vi "dfd_Cosine Modulation.vi"(6 "fs in [Hz]":dbl=1.0, 7 "number of bands":i32=4, 8 "error in (no error)":errorcluster, 11 "h":dbl[](array[numeric])) -> (0 "error out":errorcluster, 2 "synthesis bank":T1[](array[typedef]) {"mMRate_SumWl" min=1 max=32 step=1; "mMRate_InputIwl" min=1 max=32 step=1; "mMRate_GainWl" min=1 max=32 step=1; "mMRate_OutputWl" min=1 max=32 step=1; "mMRate_InputWl" min=1 max=32 step=1; "mMRate_CoefWl" min=1 max=32 step=1; "mMRate_Mode" items=["Default"=-1, "No Rate Change"=0, "Interpolation"=1, "Decimation"=2, "Interpolated"=3, "Rational"=4]}, 3 "analysis bank":T1[](array[typedef]) {"mMRate_SumWl" min=1 max=32 step=1; "mMRate_InputIwl" min=1 max=32 step=1; "mMRate_GainWl" min=1 max=32 step=1; "mMRate_OutputWl" min=1 max=32 step=1; "mMRate_InputWl" min=1 max=32 step=1; "mMRate_CoefWl" min=1 max=32 step=1; "mMRate_Mode" items=["Default"=-1, "No Rate Change"=0, "Interpolation"=1, "Decimation"=2, "Interpolated"=3, "Rational"=4]})   [LabVIEW 2017, in "NI_DigFilter_FilterBank.lvlib"]
doc: "Generates <B>analysis bank</B> and <B>synthesis bank</B> by cosine modulation of <B>prototype filter</B>."
uses:
  <vilib>/addons/Digital Filter Design/NI_DigFilter_FilterBank.lvlib
  <vilib>/addons/Digital Filter Design/_Objects.llb/DFD Multirate Filter Obj.ctl
  <vilib>/addons/Digital Filter Design/_Objects.llb/DFD Multirate Mode.ctl
  <vilib>/addons/Digital Filter Design/_Objects.llb/DFD Coef Norm Type.ctl
  <vilib>/addons/Digital Filter Design/_Objects.llb/DFD Round-off Mode.ctl
  <vilib>/addons/Digital Filter Design/_Objects.llb/DFD FXP MRate Multiply Mode.ctl
  <vilib>/Analysis/1siggen.llb/Ramp Pattern by Samples.vi
  <vilib>/addons/Digital Filter Design/NI_DigFilterLicensed.lvlib
  <vilib>/Analysis/NI_AALBase.lvlib
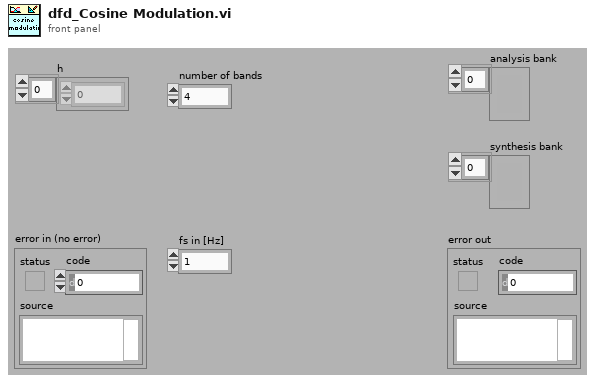
[diagram p1: front panel]
types:
  T1 = typedef "NI_DigFilterLicensed.lvlib/DFD Multirate Filter Obj.ctl" = cluster{"mMRate_Structure":enum16{"CIC", "FIR", "IIR", "Lattice"}, "mMRate_Mode":T2, "mMRate_Factor":i32, "mMRate_FIRParams":cluster{"mMRate_FIR_H":dbl[], "mMRate_FIR_IsNyquist?":bool, "mMRate_FIR_IsSymmetric?":bool}, "mMRate_CICParams":cluster{"mMRate_CIC_#Stage":i32, "mMRate_CIC_Lag":i32, "mMRate_CIC_Type":enum16{"Lowpass", "Highpass"}}, "mMRate_Order":i32, "mMRate_Version":string, "mMRate_Comments":string, "mMRate_RationalFactor":cluster{"mMRate_L":i32, "mMRate_M":i32}, "mMRate_Fs":dbl, "mMRate_Quantized?":bool, "mMRate_QFilterGain":dbl, "mMRate_CoefWl":i16, "mMRate_Scaling":cluster{"mMRate_ScaleByPowerOf2?":bool, "mMRate_ScaleType":T3}, "mMRate_InputWl":i16, "mMRate_OutputWl":i16, "mMRate_OutputMode":T4, "mMRate_MultMode":T5, "mMRate_BitPruning":bool, "mMRate_GainWl":i16, "mMRate_OutputFwl":i16, "mMRate_SumIwl":i16, "mMRate_InputIwl ":i16, "mMRate_SumWl":i16, "mMRate_CoefIwl":i16}
  T2 = typedef "NI_DigFilterLicensed.lvlib/DFD Multirate Mode.ctl" = i16
  T3 = typedef "NI_DigFilterLicensed.lvlib/DFD Coef Norm Type.ctl" = enum16{"No Norm", "Time Domain 1-Norm", "Time Domain 2-Norm", "Time Domain Inf-Norm"}
  T4 = typedef "NI_DigFilterLicensed.lvlib/DFD Round-off Mode.ctl" = enum16{"Nearest", "Truncation"}
  T5 = typedef "NI_DigFilterLicensed.lvlib/DFD FXP MRate Multiply Mode.ctl" = enum16{"Truncated", "Full"}
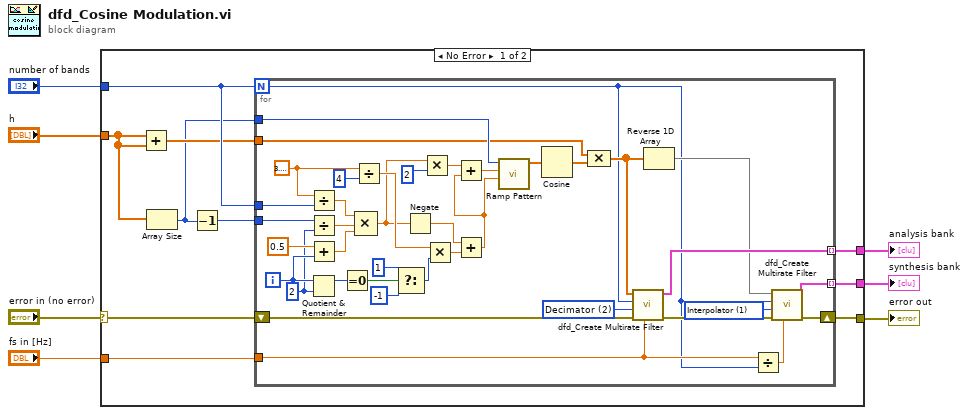
[diagram p0: block diagram]
diagram:
  n1 = case shown="No Error" "error in (no error)" {
    selector: "error in (no error)" -> [w12 w57]
    tunnel: "number of bands" -> [w17 _]
    tunnel: "h" -> [w11 _]
    tunnel: [w13 w57] -> w4
    tunnel: [w16 _] -> w3
    tunnel: [w15 _] -> w2
    tunnel: "fs in [Hz]" -> [w8 _]
    frame No Error {
      n2 = Add(x=w11, y=w11) -> (x+y=w14:dbl[])
      n3 = Array Size(array=w11) -> (size(s)=w10:i32)
      n4 = Decrement(x=w10) -> (x-1=w9:i32)
      n5 = for {
        N: w17 -> [w19]
        tunnel: w10 -> [w51]
        tunnel: w14 -> [w44]
        tunnel: w17 -> [w50]
        tunnel: w9 -> [w43]
        tunnel: [w55] -> w16 mode=indexing
        tunnel: [w24] -> w15 mode=indexing
        shift-right: [w23] -> w13
        shift-left: w12 -> [w26]
        tunnel: w8 -> [w20]
        i -> [w33]
        w21 = T2 1 items=["Default"=-1, "Normal"=0, "Interpolator"=1, "Decimator"=2, "Interpolated"=3] ("mode")
        w22 = T2 2 items=["Default"=-1, "Normal"=0, "Interpolator"=1, "Decimator"=2, "Interpolated"=3] ("mode")
        w31 = 2
        w48 = 3.141592653589793
        n6 = Divide(x=w48, y=w50) -> (x/y=w42:dbl)
        n7 = Divide(x=w43, y=w31) -> (x/y=w41:dbl)
        n8 = Add(x=0.5, y=w33) -> (x+y=w40:dbl)
        n9 = Quotient & Remainder(x=w33, y=w31) -> (x-y*floor(x/y)=w27:i32)  [unwired: 1 out]
        n10 = Equal To 0?(x=w27) -> (x = 0?=w32:bool)
        n11 = Divide(x=w48, y=4) -> (x/y=w47:dbl)
        n12 = Compound Arithmetic op=MULTIPLY(w42, w41, w40) -> (w38:dbl)
        n13 = Select(t=1, s=w32, f=-1) -> (s? t:f=w28:i32)
        n14 = Negate(x=w38) -> (-x=w46:dbl)
        n15 = Multiply(x=w38, y=2) -> (x*y=w36:dbl)
        n16 = Multiply(x=w47, y=w28) -> (x*y=w37:dbl)
        n17 = Add(x=w46, y=w37) -> (x+y=w35:dbl)
        n18 = Add(x=w36, y=w35) -> (x+y=w34:dbl)
        n19 = call-poly <vilib>:"Ramp Pattern.vi"("start"=w35, "end"=w34, "samples"=w51) -> ("Ramp Pattern"=w45:dbl[])  [unwired: 7 in, 1 out]
        n20 = Cosine(x=w45) -> (cos(x)=w52:dbl[])
        n21 = Compound Arithmetic op=MULTIPLY(w44, w52) -> (w54:dbl[])
        n22 = call <vilib>:"dfd_Create Multirate Filter.vi"("fs"=w20, "error in (no error)"=w26, "mode"=w22, "factor"=w19, "h (n)"=w54) -> ("error out"=w25:errorcluster, "multirate filter out"=w55:T1)  [unwired: 5 in]
        n23 = Reverse 1D Array(array=w54) -> (reversed array=w53:dbl[])
        n24 = Divide(x=w20, y=w19) -> (x/y=w18:dbl)
        n25 = call <vilib>:"dfd_Create Multirate Filter.vi"("fs"=w18, "error in (no error)"=w25, "mode"=w21, "factor"=w19, "h (n)"=w53) -> ("error out"=w23:errorcluster, "multirate filter out"=w24:T1)  [unwired: 5 in]
      }
    }
    frame Error {
    }
  }
  "error out" <- w4
  "analysis bank" <- w3
  "synthesis bank" <- w2
